vi "Data Width Enum to Number.vi"(0 "data width":T1) -> (4 "numberic width":u64)   [LabVIEW 2015, in "niHighSpeedSerial Eye Scan Common v1 Host.lvlib"]
uses:
  <instrlib>/niHighSpeedSerial/Eye Scan/v1/Host/Common/niHighSpeedSerial Eye Scan Common v1 Host.lvlib
  <instrlib>/niHighSpeedSerial/Eye Scan/v1/Host/Common/Public/Data Width.ctl
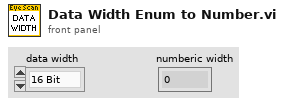
[diagram p1: front panel]
types:
  T1 = typedef "niHighSpeedSerial Eye Scan Common v1 Host.lvlib/Data Width.ctl" = enum16{"16 Bit", "20 Bit", "32 Bit", "40 Bit"}
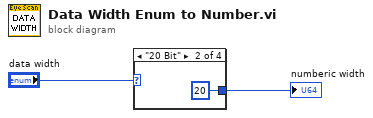
[diagram p0: block diagram]
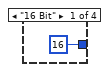
[diagram p2: hidden frame]
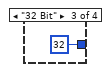
[diagram p3: hidden frame]
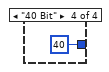
[diagram p4: hidden frame]
diagram:
  n1 = case shown="\"20 Bit\"" "data width" {
    tunnel: [u64 16 ("x") u64 20 ("x") u64 32 ("x") u64 40 ("x")] -> w1
    frame "16 Bit" {
    }
    frame "20 Bit" {
    }
    frame "32 Bit" {
    }
    frame "40 Bit" {
    }
  }
  "numberic width" <- w1
